vi "Initialize.vi"(8 "error in (no error)":errorcluster, 9 "NIVS.Gateway IP Address":string, 10 "NIVS.Workspace Event":refnum<event-registration>, 11 "State Variables":T1) -> (0 "error out":errorcluster, 3 "output cluster":T1={"CD Path"="", "CD IP"="", "Settings"={"Control Loop Names"=[], "Enable Live Updates"=[], "Gain Schedule"=[], "Enable Gain Scheduling"=[]}, "NIVS.SysDefRoot"=refnum, "NIVS.Workspace"=refnum, "NIVS.UserEvents"={"NIVS.Workspace Event"=refnum, "SystemChangeEventRef"=refnum}, "NIVS.SystemStateRefs"={"CustDatRef"=refnum, "EvtRef"=refnum, "Target State User Event"=refnum}, "UI.PIDSettingsMenu"=["Tool.Configure", "Gains.Import", "Gains.Export"], "Comm Info"={"connection ID"=refnum, "meta data"=[]}, "Addon.Connected?"=FALSE, "UI.Refs"={"Controller"=refnum, "GainSettings"=refnum, "Device"=refnum, "GainSchedulingAllowed?"=refnum, "LiveUpdatesAllowed?"=refnum, "Revert"=refnum, "Apply"=refnum}, "NIVS.SysDef"=refnum, "Data.UDPChannels"=[], "Data.Found?"=FALSE, "Data.PreviousValues"=[], "Data.SlowChannels"=[], "Data.PendingChange?"=FALSE, "Data.UDPEngineQueue"=refnum, "UI.Chart.Refs"={"Chart"=refnum, "Manual Value"=refnum, "Manual Output"=refnum, "Revert"=refnum, "Apply"=refnum, "Setpoint"=refnum, "Autoscale X"=refnum, "Autoscale Y"=refnum, "Hold"=refnum, "Manual Control"=refnum}, "Controller.SetpointRange"={"Min"=0.0, "Max"=0.0}, "Controller.OutputRange"={"Min"=0.0, "Max"=0.0}})   [LabVIEW 2019, in "Control Workspace Tool.lvlib"]
uses:
  Control Workspace Tool.lvlib
  Types/Tool State Variables.ctl
  Addon/Addon Shared/Types/Get Settings Message.ctl
  Addon/Addon Shared/Types/Gain Schedule.ctl
  NationalInstruments.VeriStand.SystemStorage
  <vilib>/NI VeriStand/Execution/Workspace/WorkspaceAPI.ctl
  NationalInstruments.VeriStand.ClientAPI
  <vilib>/NI VeriStand/Execution/Workspace/SystemStateRegEventRef.ctl
  <vilib>/NI VeriStand/Execution/Workspace/Target State Info.ctl
  <vilib>/NI VeriStand/Execution/Workspace/Target State.ctl
  <vilib>/NI VeriStand/Execution/Workspace/SystemStateEventRef.ctl
  <vilib>/NI/STM/TCP/TCP Connection Info.ctl
  <vilib>/NI/STM/SubVIs/MetaDataElement.ctl
  Types/UI Refs.ctl
  NationalInstruments.VeriStand.SystemDefinitionAPI
  Workspace Objects/Types/UDP Streaming Command Cluster.ctl
  Workspace Objects/Types/UDP Streaming State.ctl
  Workspace Objects/Types/UI.Chart.Refs.ctl
  <vilib>/NI VeriStand/Execution/Workspace/NI_VS Workspace ExecutionAPI.lvlib
  Workspace Objects/Control Workspace Object.lvlib
  Addon/Addon Shared/Control Addon Shared.lvlib
  <vilib>/NI/STM/NI STM.lvlib
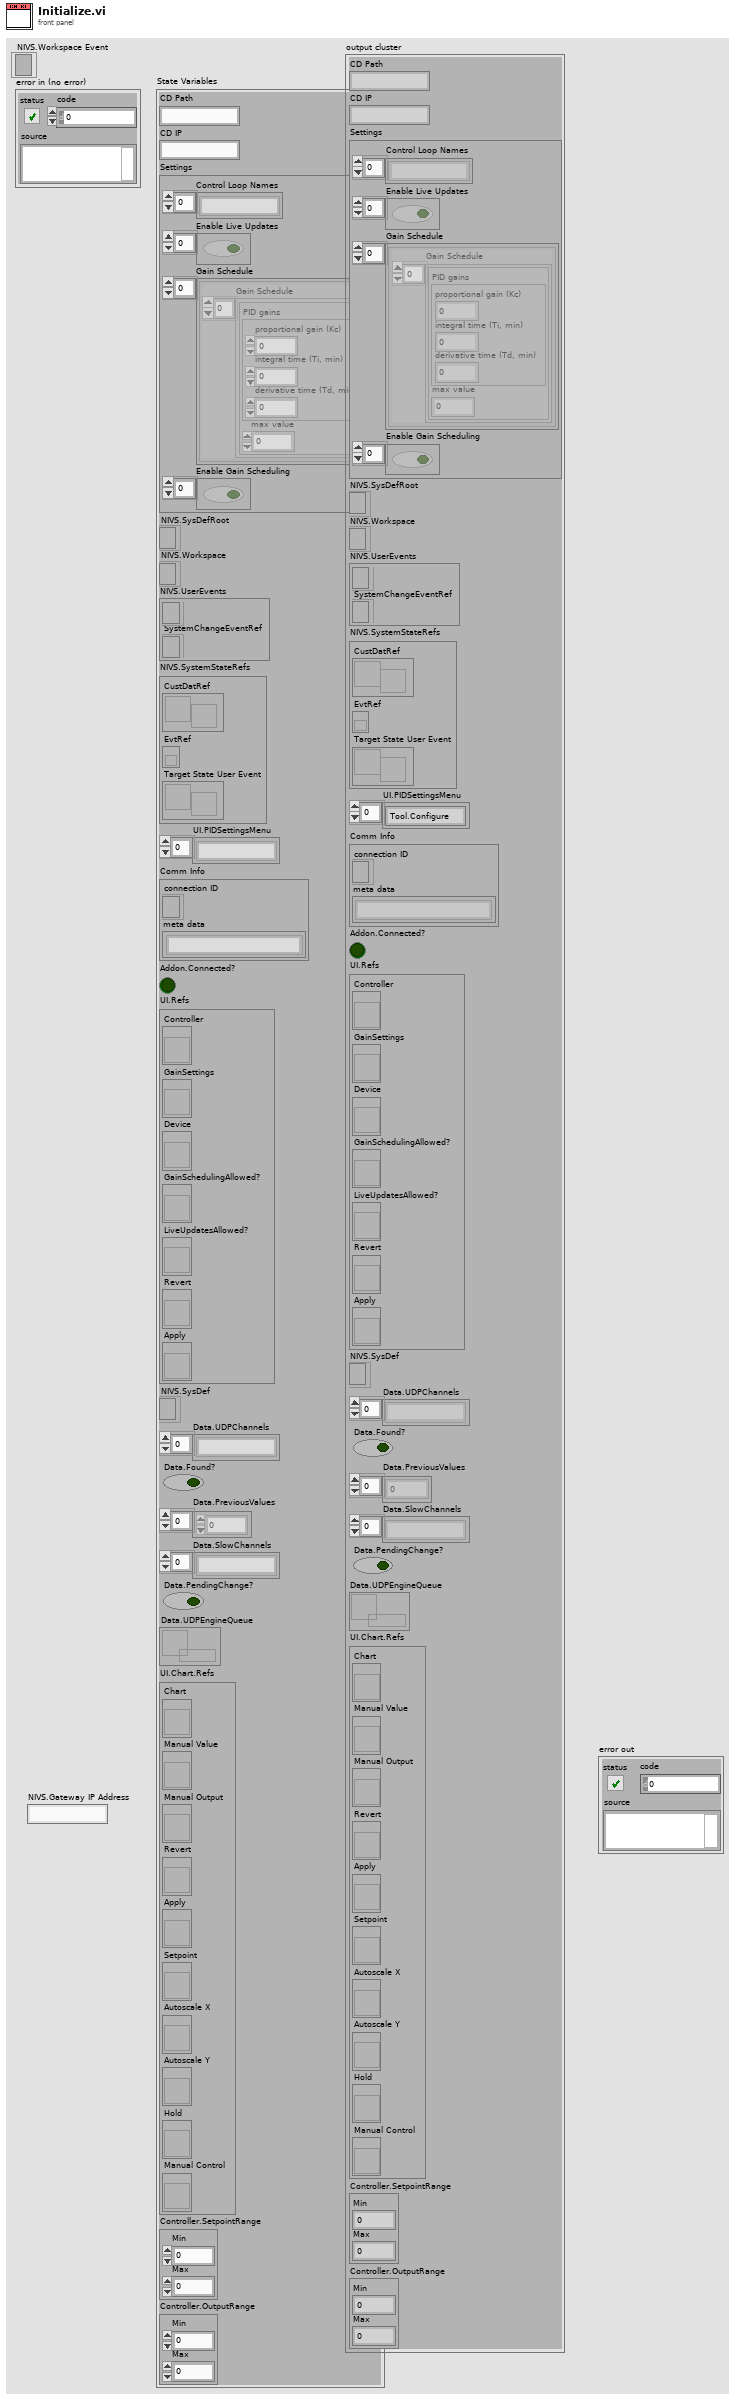
[diagram p1: front panel]
types:
  T1 = typedef "Control Workspace Tool.lvlib/Tool State Variables.ctl" = cluster{"CD Path":string, "CD IP":string, "Settings":T2, "NIVS.SysDefRoot":refnum<k24>, "NIVS.Workspace":T4, "NIVS.UserEvents":cluster{"NIVS.Workspace Event":refnum<event-registration>, "SystemChangeEventRef":T5}, "NIVS.SystemStateRefs":T6, "UI.PIDSettingsMenu":string[], "Comm Info":T7, "Addon.Connected?":bool, "UI.Refs":T9, "NIVS.SysDef":refnum<k24>, "Data.UDPChannels":string[], "Data.Found?":bool, "Data.PreviousValues":dbl[], "Data.SlowChannels":string[], "Data.PendingChange?":bool, "Data.UDPEngineQueue":refnum<queue>, "UI.Chart.Refs":T10, "Controller.SetpointRange":cluster{"Min":dbl, "Max":dbl}, "Controller.OutputRange":cluster{"Min":dbl, "Max":dbl}}
  T2 = typedef "Control Addon Shared.lvlib/Get Settings Message.ctl" = cluster{"Control Loop Names":string[], "Enable Live Updates":bool[], "Gain Schedule":T3[], "Enable Gain Scheduling":bool[]}
  T3 = typedef "Control Addon Shared.lvlib/Gain Schedule.ctl" = cluster{"Gain Schedule":cluster{"PID gains":cluster{"proportional gain (Kc)":dbl, "integral time (Ti, min)":dbl, "derivative time (Td, min)":dbl}, "max value":dbl}[]}
  T4 = typedef "NI_VS Workspace ExecutionAPI.lvlib/WorkspaceAPI.ctl" = refnum<k24>
  T5 = typedef "NI_VS Workspace ExecutionAPI.lvlib/SystemStateRegEventRef.ctl" = refnum<event-registration>
  T6 = typedef "NI_VS Workspace ExecutionAPI.lvlib/SystemStateEventRef.ctl" = cluster{"CustDatRef":refnum<user-event>, "EvtRef":refnum<k27>, "Target State User Event":refnum<user-event>}
  T7 = typedef "NI STM.lvlib/TCP Connection Info.ctl" = cluster{"connection ID":refnum<k5>, "meta data":T8[]}
  T8 = typedef "NI STM.lvlib/MetaDataElement.ctl" = string
  T9 = typedef "Control Workspace Tool.lvlib/UI Refs.ctl" = cluster{"Controller":refnum<vi>, "GainSettings":refnum<vi>, "Device":refnum<vi>, "GainSchedulingAllowed?":refnum<vi>, "LiveUpdatesAllowed?":refnum<vi>, "Revert":refnum<vi>, "Apply":refnum<vi>}
  T10 = typedef "Control Workspace Object.lvlib/UI.Chart.Refs.ctl" = cluster{"Chart":refnum<vi>, "Manual Value":refnum<vi>, "Manual Output":refnum<vi>, "Revert":refnum<vi>, "Apply":refnum<vi>, "Setpoint":refnum<vi>, "Autoscale X":refnum<vi>, "Autoscale Y":refnum<vi>, "Hold":refnum<vi>, "Manual Control":refnum<vi>}
  T11 = typedef "Control Workspace Object.lvlib/UDP Streaming Command Cluster.ctl" = cluster{"Action":T12, "Channels":string[]}
  T12 = typedef "Control Workspace Object.lvlib/UDP Streaming State.ctl" = enum8{"Idle", "Start Acq", "Run", "Stop Acq", "Exit"}
  T13 = cluster{"NIVS.Workspace Event":refnum<event-registration>, "SystemChangeEventRef":T5}
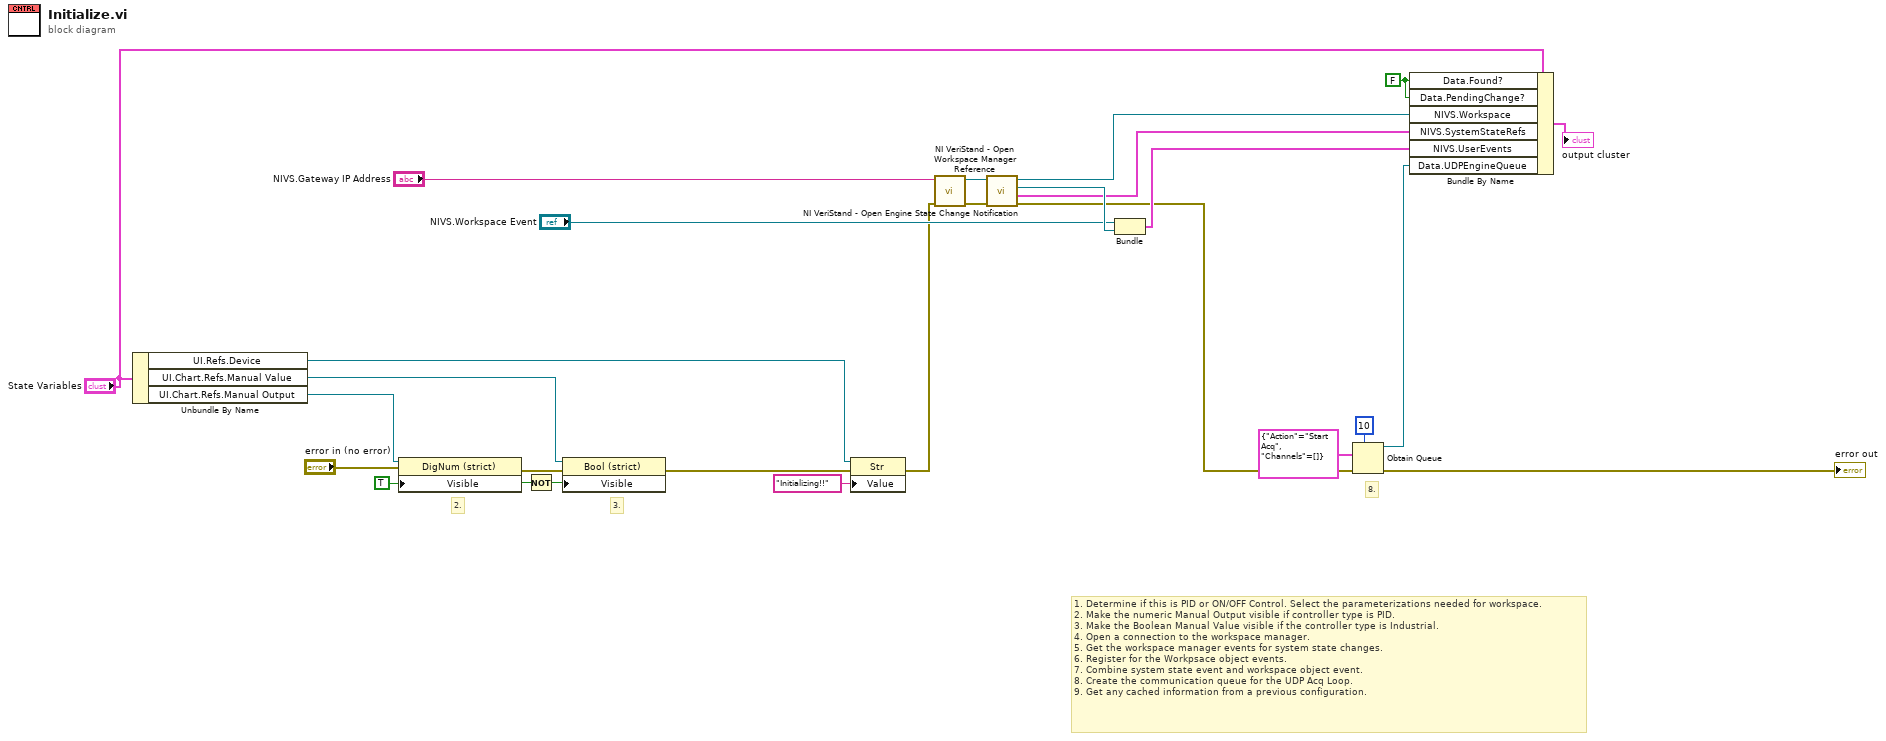
[diagram p0: block diagram]
diagram:
  w1 = FALSE ("Controller.Selected?")
  w22 = TRUE ("Visible")
  # "1. Determine if this is PID or ON/OFF Control. Select the parameterizations needed for workspace.\n2. Make the numeric Manual Output visible if controller type is PID.\n3. Make the Boolean Manual Value visible if the controller type is Industrial.\n4. Open a connection to the workspace manager.\n5. Get the workspace manager events for system state changes.\n6. Register for the Workpsace object events.\n7. Combine system state event and workspace object event.\n8. Create the communication queue for the UDP Acq Loop.\n9. Get any cached information from a previous configuration."
  # "8."
  # "3."
  # "2."
  n1 = Unbundle By Name("State Variables") -> ("UI.Refs.Device"=w2:refnum<vi>, "UI.Chart.Refs.Manual Value"=w21:refnum<vi>, "UI.Chart.Refs.Manual Output"=w23:refnum<vi>)
  n2 = property class="DigNum (strict)"(reference=w23, error in="error in (no error)", "Visible"=w22) -> (error out=w19:errorcluster)  [unwired: 1 out]
  n3 = Not(x=w22) -> (.not. x?=w20:bool)
  n4 = property class="Bool (strict)"(reference=w21, error in=w19, "Visible"=w20) -> (error out=w4:errorcluster)  [unwired: 1 out]
  n5 = property class="Str"(reference=w2, error in=w4, "Value"="Initializing!!") -> (error out=w3:errorcluster)  [unwired: 1 out]
  n6 = call <vilib>:"NI VeriStand - Open Workspace Manager Reference.vi"("error in (no error)"=w3, "Gateway IP Address (\"\": localhost)"="NIVS.Gateway IP Address") -> ("error out"=w17:errorcluster, "WorkspaceManager"=w18:T4)  [unwired: 8 in]
  n7 = call <vilib>:"NI VeriStand - Open Engine State Change Notification.vi"("error in (no error)"=w17, "WorkspaceManager in"=w18) -> ("error out"=w10:errorcluster, "SystemStateRefs"=w11:T6, "SystemChangeEventRef"=w16:T5, "WorkspaceManager out"=w15:T4)  [unwired: 6 in]
  n8 = Bundle("NIVS.Workspace Event"="NIVS.Workspace Event", "SystemChangeEventRef"=w16) -> (w14:T13)  [unwired: 1 in]
  n9 = Obtain Queue(max queue size (-1, unlimited)=10, element data type=T11 {"Action"=enum."Start Acq", "Channels"=[]}, error in (no error)=w10) -> (queue out=w9:refnum<queue>, error out=→"error out":errorcluster)  [unwired: 2 in, 1 out]
  n10 = Bundle By Name(cluster="State Variables", "Data.Found?"=w1, "Data.PendingChange?"=w1, "NIVS.Workspace"=w15, "NIVS.SystemStateRefs"=w11, "NIVS.UserEvents"=w14, "Data.UDPEngineQueue"=w9) -> (→"output cluster":T1)
